vi "To Pretty String.vi"(8 "error in (no error)":errorcluster, 11 "JSON Object in":refnum<class "JSON Object.lvclass">) -> (0 "error out":errorcluster, 3 "Pretty Print String":string)   [LabVIEW 2015, in "LVJSON.lvlib" / "JSON Object.lvclass"]
uses:
  JSON Object.lvclass
  JSON Datatype/JSON Datatype.lvclass
  LVJSON.lvlib
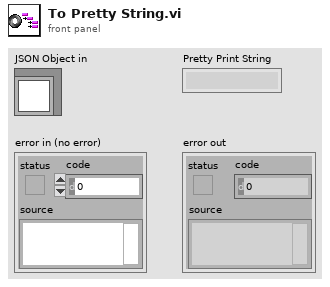
[diagram p1: front panel]
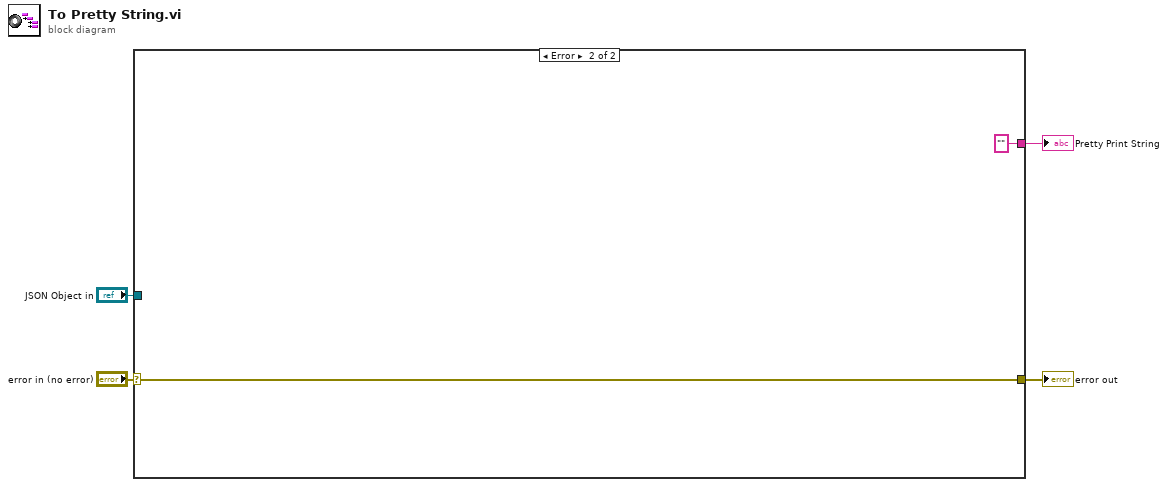
[diagram p0: block diagram]
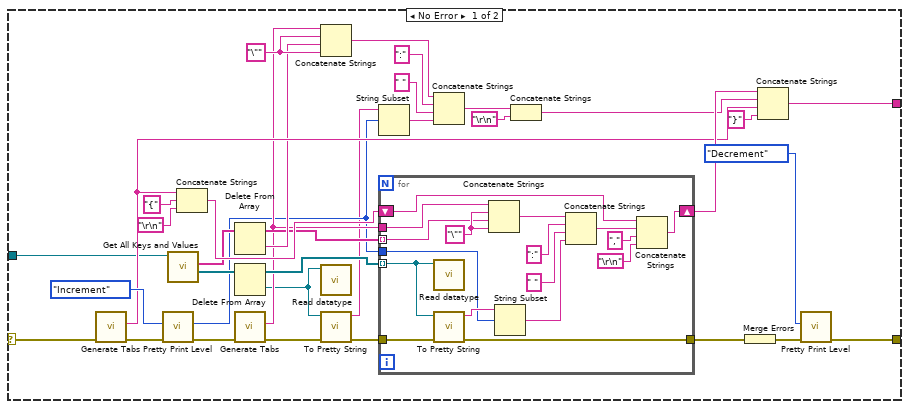
[diagram p2: hidden frame]
diagram:
  n1 = case shown="Error" "error in (no error)" {
    selector: "error in (no error)" -> [w23 w57]
    tunnel: [w25 ""] -> w4
    tunnel: [w24 w57] -> w3
    tunnel: "JSON Object in" -> [w14 _]
    frame No Error {
      w19 = "\"" ("string")
      n2 = call "Generate Tabs.vi"("error in (no error)"=w23) -> ("error out"=w36:errorcluster, "Tabs"=w26:string)  [unwired: 9 in]
      n3 = call "Pretty Print Level.vi"("error in (no error)"=w36, "Action"=enum16{"Increment", "Decrement", "Get", "Reset"}."Increment") -> ("error out"=w33:errorcluster, "Numeric"=w7:i32)  [unwired: 8 in]
      n4 = call "Get All Keys and Values.vi"("LVJSON.lvlib:JSON Object.lvclass"=w14) -> ("values"=w22:refnum<class "JSON Datatype.lvclass">[], "keys"=w21:string[])  [unwired: 8 in, 1 out]
      n5 = Concatenate Strings(w26, "{" ("string"), "\r\n") -> (w37:string)
      n6 = Delete From Array(array=w21) -> (deleted portion=w17:string, array with subset deleted=w15:string[])  [unwired: 2 in]
      n7 = Delete From Array(array=w22) -> (deleted portion=w10:refnum<class "JSON Datatype.lvclass">, array with subset deleted=w32:refnum<class "JSON Datatype.lvclass">[])  [unwired: 2 in]
      n8 = call "Generate Tabs.vi"("error in (no error)"=w33) -> ("error out"=w9:errorcluster, "Tabs"=w12:string)  [unwired: 9 in]
      n9 = Concatenate Strings(w12, w19, w17, w19) -> (w18:string)
      n10 = call-dynamic "Read datatype.vi"("JSON Datatype in"=w10) -> ()  [unwired: 8 in, 3 out]
      n11 = call-dynamic "To Pretty String.vi"("error in (no error)"=w9, "JSON Datatype in"=w10) -> ("error out"=w8:errorcluster, "Pretty Print String"=w6:string)  [unwired: 8 in]
      n12 = String Subset(string=w6, offset (0)=w7) -> (substring=w5:string)  [unwired: 1 in]
      n13 = for {
        tunnel: w32 -> [w44] mode=indexing
        shift-right: [w54] -> w30
        shift-left: w37 -> [w53]
        tunnel: w12 -> [w46]
        tunnel: w15 -> [w49] mode=indexing
        tunnel: w8 -> [w45]
        tunnel: [w43] -> w11
        tunnel: w7 -> [w41]
        w51 = "\"" ("string")
        n14 = call-dynamic "Read datatype.vi"("JSON Datatype in"=w44) -> ()  [unwired: 8 in, 3 out]
        n15 = call-dynamic "To Pretty String.vi"("error in (no error)"=w45, "JSON Datatype in"=w44) -> ("error out"=w43:errorcluster, "Pretty Print String"=w42:string)  [unwired: 8 in]
        n16 = Concatenate Strings(w46, w51, w49, w51) -> (w52:string)
        n17 = String Subset(string=w42, offset (0)=w41) -> (substring=w40:string)  [unwired: 1 in]
        n18 = Concatenate Strings(w52, ":" ("string"), " " ("string"), w40) -> (w48:string)
        n19 = Concatenate Strings(w53, w48, "," ("string"), "\r\n") -> (w54:string)
      }
      n20 = Concatenate Strings(w18, ":" ("string"), " " ("string"), w5) -> (w16:string)
      n21 = Concatenate Strings(w16, "\r\n") -> (w29:string)
      n22 = Merge Errors(w11) -> (w35:errorcluster)
      n23 = Concatenate Strings(w30, w29, w26, "}" ("string")) -> (w25:string)
      n24 = call "Pretty Print Level.vi"("error in (no error)"=w35, "Action"=enum16{"Increment", "Decrement", "Get", "Reset"}."Decrement") -> ("error out"=w24:errorcluster)  [unwired: 8 in, 1 out]
    }
    frame Error {
    }
  }
  "error out" <- w3
  "Pretty Print String" <- w4
